vi "scale_names_match.vi"(10 "Last Axis output cluster":T1, 11 "Axis output cluster":T1) -> (3 "result":bool)   [LabVIEW 2020, in "3DPC_SurfacePlot.xctl"]
uses:
  <vilib>/Native 3D Graph/xcontrol/3DPC_SurfacePlot.xctl
  <vilib>/Native 3D Graph/typedefs/prop_axes_merged_array_etc.ctl
  <vilib>/Native 3D Graph/typedefs/prop_axes_merged_array.ctl
  <vilib>/Native 3D Graph/typedefs/range_cluster.ctl
  <vilib>/Native 3D Graph/typedefs/min_max.ctl
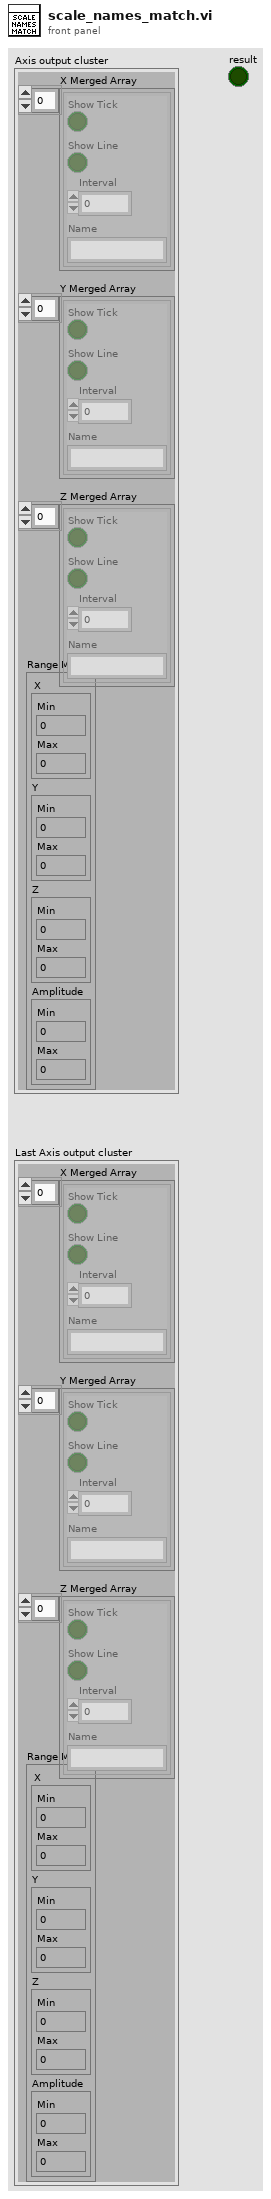
[diagram p1: front panel]
types:
  T1 = typedef "3DPC_SurfacePlot.xctl/prop_axes_merged_array_etc.ctl" = cluster{"X Merged Array":T2, "Y Merged Array":T2, "Z Merged Array":T2, "Range Min/Max":T3}
  T2 = typedef "3DPC_SurfacePlot.xctl/prop_axes_merged_array.ctl" = cluster{"Show Tick":bool, "Show Line":bool, "Interval":sgl, "Name":string}[]
  T3 = typedef "3DPC_SurfacePlot.xctl/range_cluster.ctl" = cluster{"X":T4, "Y":T4, "Z":T4, "Amplitude":T4}
  T4 = typedef "3DPC_SurfacePlot.xctl/min_max.ctl" = cluster{"Min":sgl, "Max":sgl}
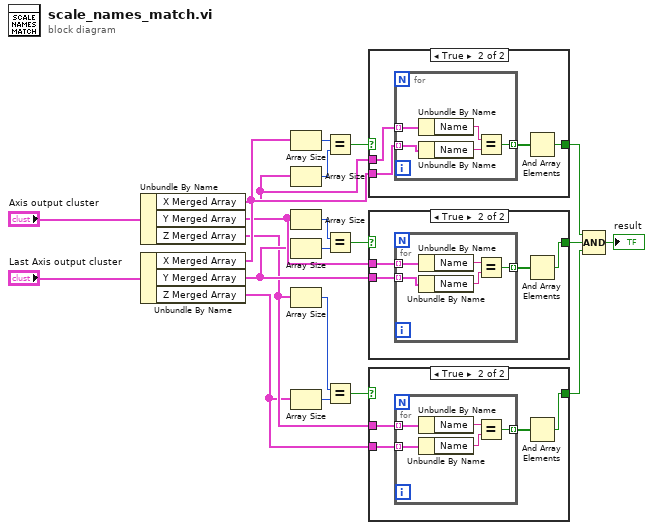
[diagram p0: block diagram]
diagram:
  n1 = Unbundle By Name("Axis output cluster") -> ("X Merged Array"=w12:T2, "Y Merged Array"=w8:T2, "Z Merged Array"=w3:T2)
  n2 = Unbundle By Name("Last Axis output cluster") -> ("X Merged Array"=w15:T2, "Y Merged Array"=w7:T2, "Z Merged Array"=w2:T2)
  n3 = Array Size(array=w15) -> (size(s)=w14:i32)
  n4 = Array Size(array=w12) -> (size(s)=w13:i32)
  n5 = Array Size(array=w8) -> (size(s)=w9:i32)
  n6 = Array Size(array=w7) -> (size(s)=w10:i32)
  n7 = Array Size(array=w3) -> (size(s)=w5:i32)
  n8 = Array Size(array=w2) -> (size(s)=w4:i32)
  n9 = Equal?(x=w14, y=w13) -> (x = y?=w11:bool)
  n10 = Equal?(x=w9, y=w10) -> (x = y?=w6:bool)
  n11 = Equal?(x=w5, y=w4) -> (x = y?=w1:bool)
  n12 = case shown="True" w11 {
    selector: w11 -> [w22 _]
    tunnel: [w22 w25] -> w19
    tunnel: w15 -> [_ w24]
    tunnel: w12 -> [_ w23]
    frame False {
    }
    frame True {
      n13 = for {
        tunnel: w23 -> [w31] mode=indexing
        tunnel: w24 -> [w30] mode=indexing
        tunnel: [w27] -> w26 mode=indexing
        n14 = Unbundle By Name(w31) -> ("Name"=w29:string)
        n15 = Unbundle By Name(w30) -> ("Name"=w28:string)
        n16 = Equal?(x=w29, y=w28) -> (x = y?=w27:bool)
      }
      n17 = And Array Elements(Boolean array=w26) -> (logical AND=w25:bool)
    }
  }
  n18 = case shown="True" w6 {
    selector: w6 -> [w32 _]
    tunnel: [w32 w35] -> w18
    tunnel: w8 -> [_ w34]
    tunnel: w7 -> [_ w33]
    frame False {
    }
    frame True {
      n19 = for {
        tunnel: w34 -> [w41] mode=indexing
        tunnel: w33 -> [w40] mode=indexing
        tunnel: [w37] -> w36 mode=indexing
        n20 = Unbundle By Name(w41) -> ("Name"=w39:string)
        n21 = Unbundle By Name(w40) -> ("Name"=w38:string)
        n22 = Equal?(x=w39, y=w38) -> (x = y?=w37:bool)
      }
      n23 = And Array Elements(Boolean array=w36) -> (logical AND=w35:bool)
    }
  }
  n24 = case shown="True" w1 {
    selector: w1 -> [w42 _]
    tunnel: w2 -> [_ w46]
    tunnel: w3 -> [_ w45]
    tunnel: [w42 w43] -> w17
    frame False {
    }
    frame True {
      n25 = for {
        tunnel: w45 -> [w51] mode=indexing
        tunnel: w46 -> [w50] mode=indexing
        tunnel: [w47] -> w44 mode=indexing
        n26 = Unbundle By Name(w51) -> ("Name"=w49:string)
        n27 = Unbundle By Name(w50) -> ("Name"=w48:string)
        n28 = Equal?(x=w49, y=w48) -> (x = y?=w47:bool)
      }
      n29 = And Array Elements(Boolean array=w44) -> (logical AND=w43:bool)
    }
  }
  n30 = Compound Arithmetic op=AND(w19, w18, w17) -> (→"result":bool)
